vi "FPGA_controller.vi"() -> ()   [LabVIEW 2017]
uses:
  <vilib>/rvi/Emulation/niFpgaGetClockAttributes.vi
  <vilib>/rvi/Emulation/niFpgaSctlEmulationGetInTimedLoop.vi
  <vilib>/rvi/Emulation/niFpgaEmulationReportErrorSimple.vi
  <vilib>/rvi/eio/common/nirviEmuTemplateMethod_errors.vi
  <vilib>/rvi/Emulation/niFpgaCriticalErrorInLSC.vi
  <vilib>/eio/EIONode/EIONode.xnode
panel:
  out "VALID":bool
  in  "m_first u2":fxp<+/-,64,32>=-0.8999999999068677 format="%#_42g"
  in  "m_first u1":fxp<+/-,64,32>=-0.8999999999068677 format="%#_42g"
  in  "Scale u2":fxp<+/-,64,42>=5.0 format="%#_35g"
  in  "Offset u2":fxp<+/-,64,41>=2.0 format="%#_36g"
  in  "Scale u1":fxp<+/-,64,42>=5.0 format="%#_35g"
  in  "Offset u1":fxp<+/-,64,41>=2.0 format="%#_36g"
  in  "eta u":fxp<+/-,64,32>=0.30000000004656613 format="%#_42g"
  in  "Scale x2":fxp<+/-,32,16>=10.0 format="%#_21g"
  in  "m_first x2":fxp<+/-,49,33> format="%#_26g"
  in  "Offset x2":fxp<+/-,48,32> format="%#_26g"
  in  "Offset x3":fxp<+/-,48,32>=5.0 format="%#_26g"
  in  "m_first x3":fxp<+/-,32,16>=-3.399993896484375 format="%#_21g"
  in  "Scale x3":fxp<+/-,32,16>=10.0 format="%#_21g"
  in  "1/eta x":fxp<+/-,32,16>=5.0 format="%#_21g"
  in  "m_first x1":fxp<+/-,49,33> format="%#_26g"
  in  "Offset x1":fxp<+/-,48,32> format="%#_26g"
  in  "Scale x1":fxp<+/-,32,16>=10.0 format="%#_21g"
  in  "stop":bool
  # "INPUTS CONVERSION"
  # "STATES CONVERSION"
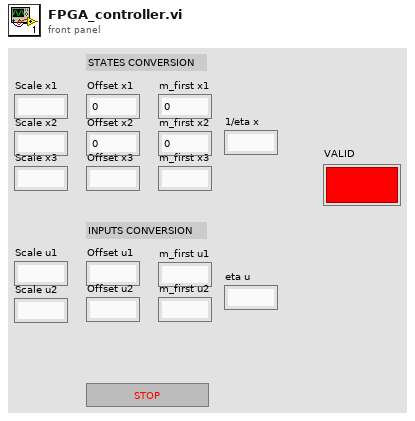
[diagram p1: front panel]
types:
  T1 = cluster{"Boolean array[0]":bool, "Boolean array[1]":bool, "Boolean array[2]":bool, "Boolean array[3]":bool, "Boolean array[4]":bool, "Boolean array[5]":bool, "Boolean array[6]":bool, "Boolean array[7]":bool, "Boolean array[8]":bool, "Boolean array[9]":bool, "Boolean array[10]":bool, "Boolean array[11]":bool, "Boolean array[12]":bool, "Boolean array[13]":bool, "Boolean array[14]":bool, "Boolean array[15]":bool, "Boolean array[16]":bool, "Boolean array[17]":bool}
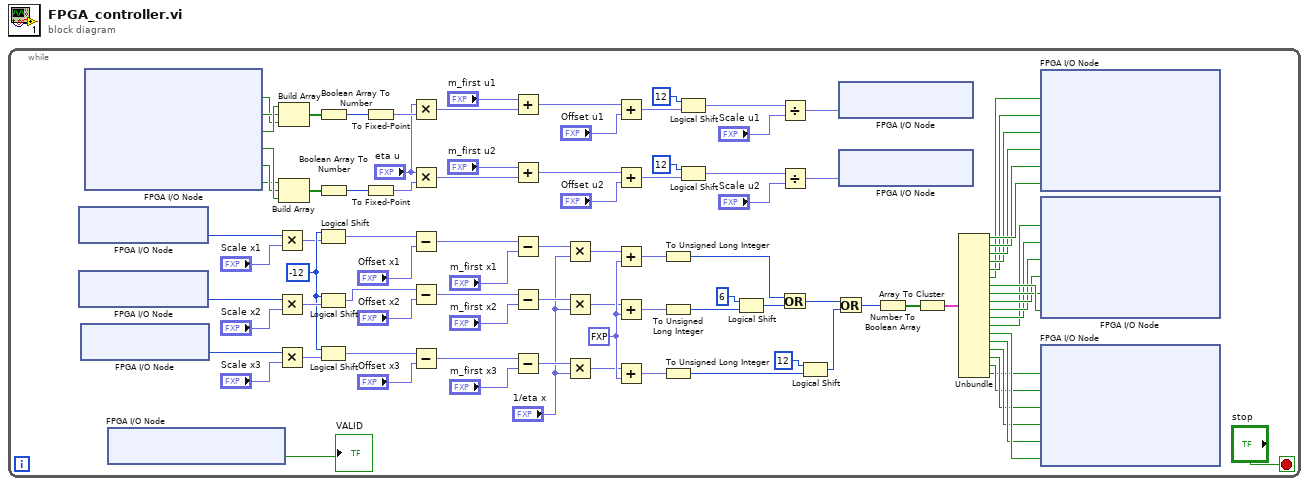
[diagram p0: block diagram]
diagram:
  n1 = while {
    stop <- "stop" stop-if-true
    w35 = fxp<+/-,64,32> 0.5 ("y")
    w28 = i16 -12 ("y")
    n2 = xnode "FPGA I/O Node"() -> ("ConnectorA/AI0"=w17:u16)  [unwired: 1 in, 1 out]
    n3 = xnode "FPGA I/O Node"() -> ("ConnectorA/AI1"=w27:u16)  [unwired: 1 in, 1 out]
    n4 = xnode "FPGA I/O Node"() -> ("ConnectorB/AI0"=w26:u16)  [unwired: 1 in, 1 out]
    n5 = xnode "FPGA I/O Node"() -> ("Component-Level IP\\po0"=w92:bool, "Component-Level IP\\po1"=w93:bool, "Component-Level IP\\po2"=w94:bool, "Component-Level IP\\po3"=w69:bool, "Component-Level IP\\po4"=w68:bool, "Component-Level IP\\po5"=w67:bool)  [unwired: 6 in, 6 out]
    n6 = xnode "FPGA I/O Node"() -> ("Component-Level IP\\po6"=→"VALID":bool)  [unwired: 1 in, 1 out]
    n7 = Multiply(x=w17, y="Scale x1") -> (x*y=w16:fxp<+/-,48,32>)
    n8 = Multiply(x=w27, y="Scale x2") -> (x*y=w37:fxp<+/-,48,32>)
    n9 = Multiply(x=w26, y="Scale x3") -> (x*y=w23:fxp<+/-,48,32>)
    n10 = Build Array(w94, w93, w92) -> (w90:bool[])
    n11 = Build Array(w67, w68, w69) -> (w78:bool[])
    n12 = Logical Shift(y=w28, x=w16) -> (x << y=w12:fxp<+/-,48,32>)
    n13 = Logical Shift(y=w28, x=w37) -> (x << y=w6:fxp<+/-,48,32>)
    n14 = Logical Shift(y=w28, x=w23) -> (x << y=w22:fxp<+/-,48,32>)
    n15 = Boolean Array To Number(Boolean array=w90) -> (number=w86:u8)
    n16 = Boolean Array To Number(Boolean array=w78) -> (number=w75:u8)
    n17 = To Fixed-Point(number=w86) -> (fixed-point=w85:fxp<+,8,8>)  [unwired: 1 in]
    n18 = To Fixed-Point(number=w75) -> (fixed-point=w74:fxp<+,8,8>)  [unwired: 1 in]
    n19 = Multiply(x="eta u", y=w85) -> (x*y=w91:fxp<+/-,64,40>)
    n20 = Multiply(x="eta u", y=w74) -> (x*y=w79:fxp<+/-,64,40>)
    n21 = Subtract(x=w12, y="Offset x1") -> (x-y=w13:fxp<+/-,49,33>)
    n22 = Subtract(x=w6, y="Offset x2") -> (x-y=w8:fxp<+/-,49,33>)
    n23 = Subtract(x=w22, y="Offset x3") -> (x-y=w24:fxp<+/-,49,33>)
    n24 = Add(x="m_first u1", y=w91) -> (x+y=w89:fxp<+/-,64,41>)
    n25 = Add(x="m_first u2", y=w79) -> (x+y=w77:fxp<+/-,64,41>)
    n26 = Subtract(x=w13, y="m_first x1") -> (x-y=w15:fxp<+/-,50,34>)
    n27 = Subtract(x=w8, y="m_first x2") -> (x-y=w5:fxp<+/-,50,34>)
    n28 = Subtract(x=w24, y="m_first x3") -> (x-y=w32:fxp<+/-,50,34>)
    n29 = Multiply(x=w15, y="1/eta x") -> (x*y=w10:fxp<+/-,64,49>)
    n30 = Multiply(x=w5, y="1/eta x") -> (x*y=w3:fxp<+/-,64,49>)
    n31 = Multiply(x=w32, y="1/eta x") -> (x*y=w31:fxp<+/-,64,49>)
    n32 = Add(x=w89, y="Offset u1") -> (x+y=w84:fxp<+/-,64,42>)
    n33 = Add(x=w77, y="Offset u2") -> (x+y=w73:fxp<+/-,64,42>)
    n34 = Add(x=w10, y=w35) -> (x+y=w46:fxp<+/-,64,50>)
    n35 = Add(x=w3, y=w35) -> (x+y=w34:fxp<+/-,64,50>)
    n36 = Add(x=w31, y=w35) -> (x+y=w33:fxp<+/-,64,50>)
    n37 = To Unsigned Long Integer(number=w46) -> (unsigned 32bit integer=w42:u32)
    n38 = To Unsigned Long Integer(number=w34) -> (unsigned 32bit integer=w44:u32)
    n39 = To Unsigned Long Integer(number=w33) -> (unsigned 32bit integer=w40:u32)
    n40 = Logical Shift(y=i16 12, x=w84) -> (x << y=w82:fxp<+/-,64,42>)
    n41 = Logical Shift(y=i16 12, x=w73) -> (x << y=w71:fxp<+/-,64,42>)
    n42 = Logical Shift(y=6, x=w44) -> (x << y=w43:u32)
    n43 = Divide(x=w82, y="Scale u1") -> (x/y=w80:fxp<+/-,64,65>)
    n44 = Divide(x=w71, y="Scale u2") -> (x/y=w70:fxp<+/-,64,65>)
    n45 = Or(x=w42, y=w43) -> (x .or. y?=w38:u32)
    n46 = Logical Shift(y=12, x=w40) -> (x << y=w39:u32)
    n47 = Or(x=w38, y=w39) -> (x .or. y?=w21:u32)
    n48 = xnode "FPGA I/O Node"("ConnectorB/AO0"=w80) -> ()  [unwired: 1 in, 1 out]
    n49 = xnode "FPGA I/O Node"("ConnectorB/AO1"=w70) -> ()  [unwired: 1 in, 1 out]
    n50 = Number To Boolean Array(number=w21) -> (Boolean array=w47:bool[])
    n51 = Array To Cluster(array=w47) -> (cluster=w66:T1)
    n52 = Unbundle(w66) -> ("Boolean array[0]"=w65:bool, "Boolean array[1]"=w64:bool, "Boolean array[2]"=w63:bool, "Boolean array[3]"=w62:bool, "Boolean array[4]"=w61:bool, "Boolean array[5]"=w60:bool, "Boolean array[6]"=w59:bool, "Boolean array[7]"=w58:bool, "Boolean array[8]"=w57:bool, "Boolean array[9]"=w56:bool, "Boolean array[10]"=w55:bool, "Boolean array[11]"=w54:bool, "Boolean array[12]"=w53:bool, "Boolean array[13]"=w52:bool, "Boolean array[14]"=w51:bool, "Boolean array[15]"=w50:bool, "Boolean array[16]"=w49:bool, "Boolean array[17]"=w48:bool)
    n53 = xnode "FPGA I/O Node"("Component-Level IP\\pi00"=w60, "Component-Level IP\\pi01"=w61, "Component-Level IP\\pi02"=w62, "Component-Level IP\\pi03"=w63, "Component-Level IP\\pi04"=w64, "Component-Level IP\\pi05"=w65) -> ()  [unwired: 6 in, 6 out]
    n54 = xnode "FPGA I/O Node"("Component-Level IP\\pi06"=w54, "Component-Level IP\\pi07"=w55, "Component-Level IP\\pi08"=w56, "Component-Level IP\\pi09"=w57, "Component-Level IP\\pi10"=w58, "Component-Level IP\\pi11"=w59) -> ()  [unwired: 6 in, 6 out]
    n55 = xnode "FPGA I/O Node"("Component-Level IP\\pi12"=w48, "Component-Level IP\\pi13"=w49, "Component-Level IP\\pi14"=w50, "Component-Level IP\\pi15"=w51, "Component-Level IP\\pi16"=w52, "Component-Level IP\\pi17"=w53) -> ()  [unwired: 6 in, 6 out]
  }
